vi "readFromXML.vi"(8 "error in (no error)":errorcluster, 10 "XML in":string="<Declination>\n<degreesDec>46</degreesDec>\n<minutesArc>31</minutesArc>\n<secondsArc>16</secondsArc>\n</Declination>", 11 "Declination in":refnum<class "Declination.lvclass">) -> (0 "error out":errorcluster, 3 "Declination out":refnum<class "Declination.lvclass">)   [LabVIEW 2014, in "TCSDataDefinitions.lvlib" / "TCSCommand.lvlib" / "TargetConfiguration.lvlib" / "Target.lvlib" / "FixedTarget.lvlib" / "Declination.lvclass"]
uses:
  Declination.lvclass
  <userlib>/Common/UnitsAndXML/FlattenItemWithUnitToXML/FlattenPlaneAngleToXML/PlaneAngleUnit.ctl
  Declination.lvclass/Declination.ctl
  <userlib>/Common/UnitsAndXML/UnitsAndXML.lvlib
  <userlib>/Common/XML/XMLParser/XMLParser.lvclass
panel:
  out "secondsArc":dbl[unit]=7.757018897752576e-05
  out "minutesArc":dbl[unit]=0.00901753446863737
  out "degreesDec":dbl[unit]=0.8028514559173916
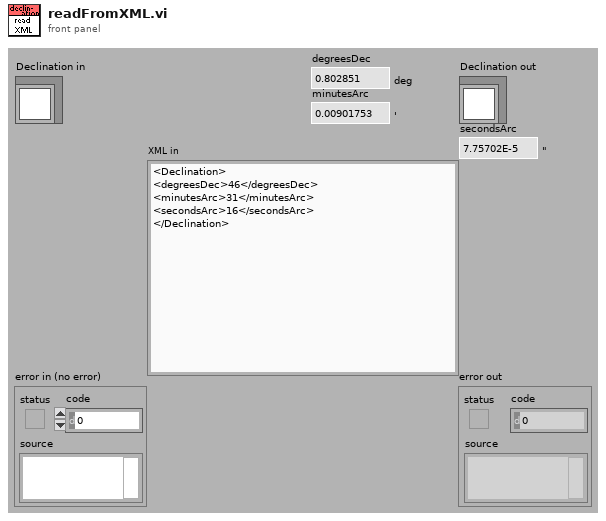
[diagram p1: front panel]
types:
  T1 = typedef "UnitsAndXML.lvlib/PlaneAngleUnit.ctl" = enum16{"rad", "deg", "'", "\""}
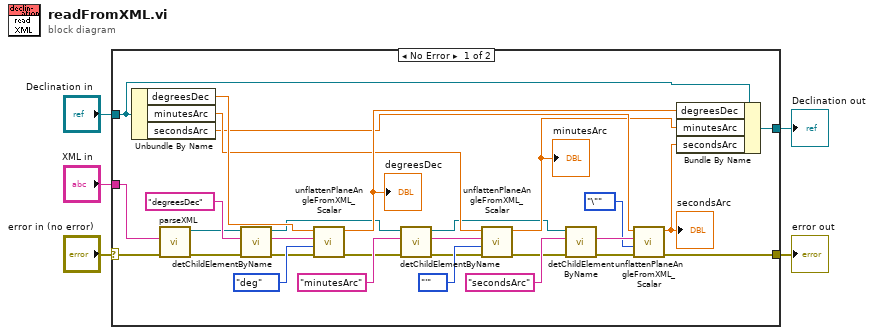
[diagram p0: block diagram]
diagram:
  n1 = case shown="No Error" "error in (no error)" {
    selector: "error in (no error)" -> [w33 w36]
    tunnel: [w11 w36] -> w4
    tunnel: [w23 w35] -> w2
    tunnel: "Declination in" -> [w24 w35]
    tunnel: "XML in" -> [w34 _]
    frame No Error {
      n2 = Unbundle By Name(w24) -> ("degreesDec"=w28:dbl[unit], "minutesArc"=w21:dbl[unit], "secondsArc"=w13:dbl[unit])
      n3 = call <userlib>:"parseXML.vi"("error in (no error)"=w33, "XMLString in"=w34) -> ("error out"=w29:errorcluster, "Element out"=w8:refnum<class "XMLParser.lvclass">)  [unwired: 8 in]
      n4 = call <userlib>:"detChildElementByName.vi"("error in (no error)"=w29, "childName"="degreesDec" ("ChildName"), "Element in"=w8) -> ("error out"=w25:errorcluster, "childXML"=w27:string, "Element out"=w7:refnum<class "XMLParser.lvclass">)  [unwired: 5 in, 1 out]
      n5 = call <userlib>:"unflattenPlaneAngleFromXML_Scalar.vi"("error in (no error)"=w25, "planeAngleUnitInXML"=PlaneAngleUnit."deg", "xmlString"=w27, "planeAngleForType"=w28) -> ("error out"=w17:errorcluster, "planeAngle"=w22:dbl[unit])  [unwired: 6 in]
      "degreesDec" <- w22
      n6 = call <userlib>:"detChildElementByName.vi"("error in (no error)"=w17, "childName"="minutesArc" ("ChildName"), "Element in"=w7) -> ("error out"=w18:errorcluster, "childXML"=w20:string, "Element out"=w6:refnum<class "XMLParser.lvclass">)  [unwired: 5 in, 1 out]
      n7 = call <userlib>:"unflattenPlaneAngleFromXML_Scalar.vi"("error in (no error)"=w18, "planeAngleUnitInXML"=PlaneAngleUnit."'", "xmlString"=w20, "planeAngleForType"=w21) -> ("error out"=w16:errorcluster, "planeAngle"=w12:dbl[unit])  [unwired: 6 in]
      "minutesArc" <- w12
      n8 = call <userlib>:"detChildElementByName.vi"("error in (no error)"=w16, "childName"="secondsArc" ("ChildName"), "Element in"=w6) -> ("error out"=w15:errorcluster, "childXML"=w14:string)  [unwired: 5 in, 2 out]
      n9 = call <userlib>:"unflattenPlaneAngleFromXML_Scalar.vi"("error in (no error)"=w15, "planeAngleUnitInXML"=PlaneAngleUnit."\"", "xmlString"=w14, "planeAngleForType"=w13) -> ("error out"=w11:errorcluster, "planeAngle"=w10:dbl[unit])  [unwired: 6 in]
      "secondsArc" <- w10
      n10 = Bundle By Name(cluster=w24, "degreesDec"=w22, "minutesArc"=w12, "secondsArc"=w10) -> (w23:refnum<class "Declination.lvclass">)
    }
    frame Error {
    }
  }
  "error out" <- w4
  "Declination out" <- w2
